vi "Configure Analog Inputs.vi"(0 "VISA resource name":refnum<visa-resource-name>, 1 "Coupling (0: cplAC)":u16(ring) items=["cplAC", "cplDC"], 2 "Range (0)":i32, 3 "Zin (0: aiHiZ)":i32(ring) items=["aiHiZ", "aiz300", "aiz600"], 5 "Channel (0: ChannelA)":i32(ring) items=["ChannelA", "ChannelB"], 7 "Hi-Res Sample Rate (0: srHz64k)":i32(ring) items=["srHz64k", "srHz128k", "srOSR", "srOSRx2"], 9 "Auto Range (T: Enable)":bool=TRUE, 11 "error in (no error)":errorcluster, 12 "Optional Filter (0: ifNone)":i32(ring) items=["ifNone", "ifFiler1", "ifFilter2", "ifFilter3", "ifFilter4", "ifGround"], 13 "Source (0: aiXLR)":i32(ring) items=["aiXLR", "aiBNC", "aiGenMon", "aiDigCommonMode"]) -> (4 "VISA resource name out":refnum<visa-resource-name>, 15 "error out":errorcluster)   [LabVIEW 2014, in "Stanford Research SR1.lvlib"]
doc: "Configures the basic attributes for the Analog Inputs."
uses:
  Stanford Research SR1.lvlib
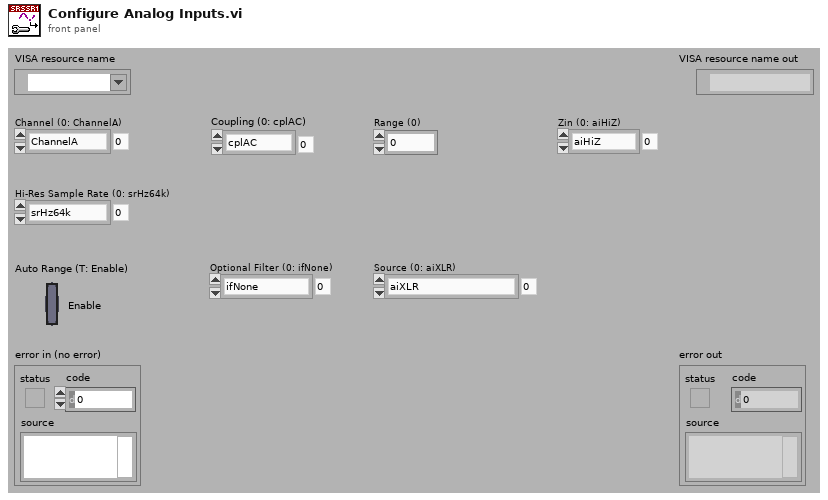
[diagram p1: front panel]
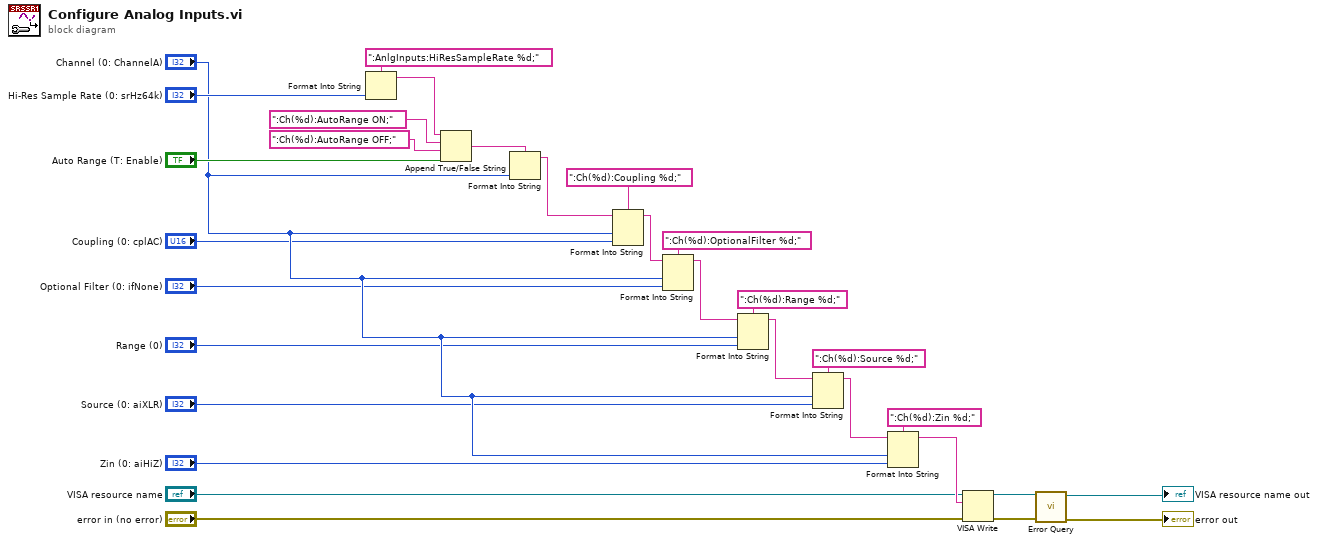
[diagram p0: block diagram]
diagram:
  n1 = Format Into String(format string=":AnlgInputs:HiResSampleRate %d;", "Hi-Res Sample Rate (0: srHz64k)") -> (resulting string=w28:string)  [unwired: 2 in, 1 out]
  n2 = Append True/False String(1:"Auto Range (T: Enable)", 2:":Ch(%d):AutoRange OFF;", 3:":Ch(%d):AutoRange ON;", 4:w28) -> (0:w14:string)
  n3 = Format Into String(format string=w14, "Channel (0: ChannelA)") -> (resulting string=w2:string)  [unwired: 2 in, 1 out]
  n4 = Format Into String(format string=":Ch(%d):Coupling %d;", initial string=w2, "Channel (0: ChannelA)", "Coupling (0: cplAC)") -> (resulting string=w13:string)  [unwired: 1 in, 1 out]
  n5 = Format Into String(format string=":Ch(%d):OptionalFilter %d;", initial string=w13, "Channel (0: ChannelA)", "Optional Filter (0: ifNone)") -> (resulting string=w23:string)  [unwired: 1 in, 1 out]
  n6 = Format Into String(format string=":Ch(%d):Range %d;", initial string=w23, "Channel (0: ChannelA)", "Range (0)") -> (resulting string=w21:string)  [unwired: 1 in, 1 out]
  n7 = Format Into String(format string=":Ch(%d):Source %d;", initial string=w21, "Channel (0: ChannelA)", "Source (0: aiXLR)") -> (resulting string=w19:string)  [unwired: 1 in, 1 out]
  n8 = Format Into String(format string=":Ch(%d):Zin %d;", initial string=w19, "Channel (0: ChannelA)", "Zin (0: aiHiZ)") -> (resulting string=w17:string)  [unwired: 1 in, 1 out]
  n9 = VISA Write(VISA resource name="VISA resource name", write buffer=w17, error in (no error)="error in (no error)") -> (VISA resource name out=w7:refnum<visa-resource-name>, error out=w6:errorcluster)  [unwired: 1 out]
  n10 = call "Error Query.vi"("error in (no error)"=w6, "VISA resource name"=w7) -> ("error out"=→"error out":errorcluster, "VISA resource name out"=→"VISA resource name out":refnum<visa-resource-name>)  [unwired: 6 in, 2 out]
